vi "BS1201 Discovery Parser.vi"(10 "IP Address":string, 11 "Discovery String":string) -> (3 "Devices":T1[](array[typedef]))   [LabVIEW 2021, in "BS120x Driver.lvlib"]
uses:
  BS120x Driver.lvlib
  New BS120x Device/DiscoveredDevice.ctl
  TypeDefs/UnitType.ctl
  TypeDefs/Protocol.ctl
  BS120x.lvclass
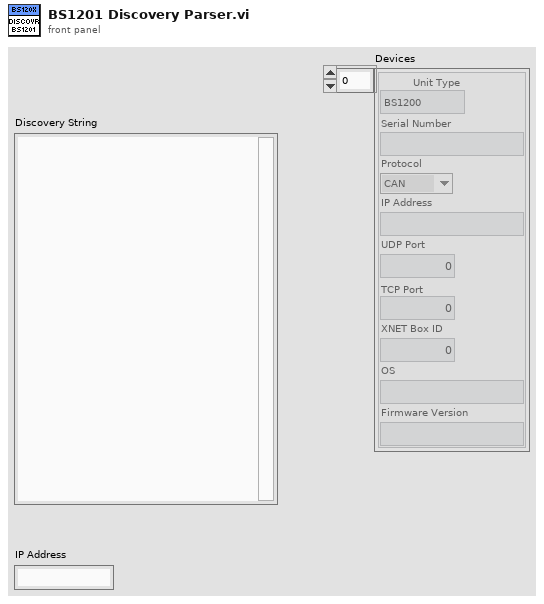
[diagram p1: front panel]
types:
  T1 = typedef "BS120x Driver.lvlib/DiscoveredDevice.ctl" = cluster{"Unit Type":T2, "Serial Number":string, "Protocol":T3, "IP Address":string, "UDP Port":u16, "TCP Port":u16, "XNET Box ID":u8, "OS":string, "Firmware Version":string}
  T2 = typedef "BS120x Driver.lvlib/BS120x.lvclass/UnitType.ctl" = enum16{"BS1200", "BS1201"}
  T3 = typedef "BS120x Driver.lvlib/BS120x.lvclass/Protocol.ctl" = enum16{"CAN", "Ethernet"}
  T4 = cluster{"IP Address":string, "SN":string, "IP Enabled":string, "UDP Port":string, "TCP Port":string, "Box ID":string}
  T5 = cluster{"IP Address":string, "SN":string, "IP Enabled":bool, "UDP Port":u16, "TCP Port":u16, "Box ID":u8}
  T6 = cluster{"[0]":string, "[1]":string, "[2]":string, "[3]":string, "[4]":string, "[5]":string}
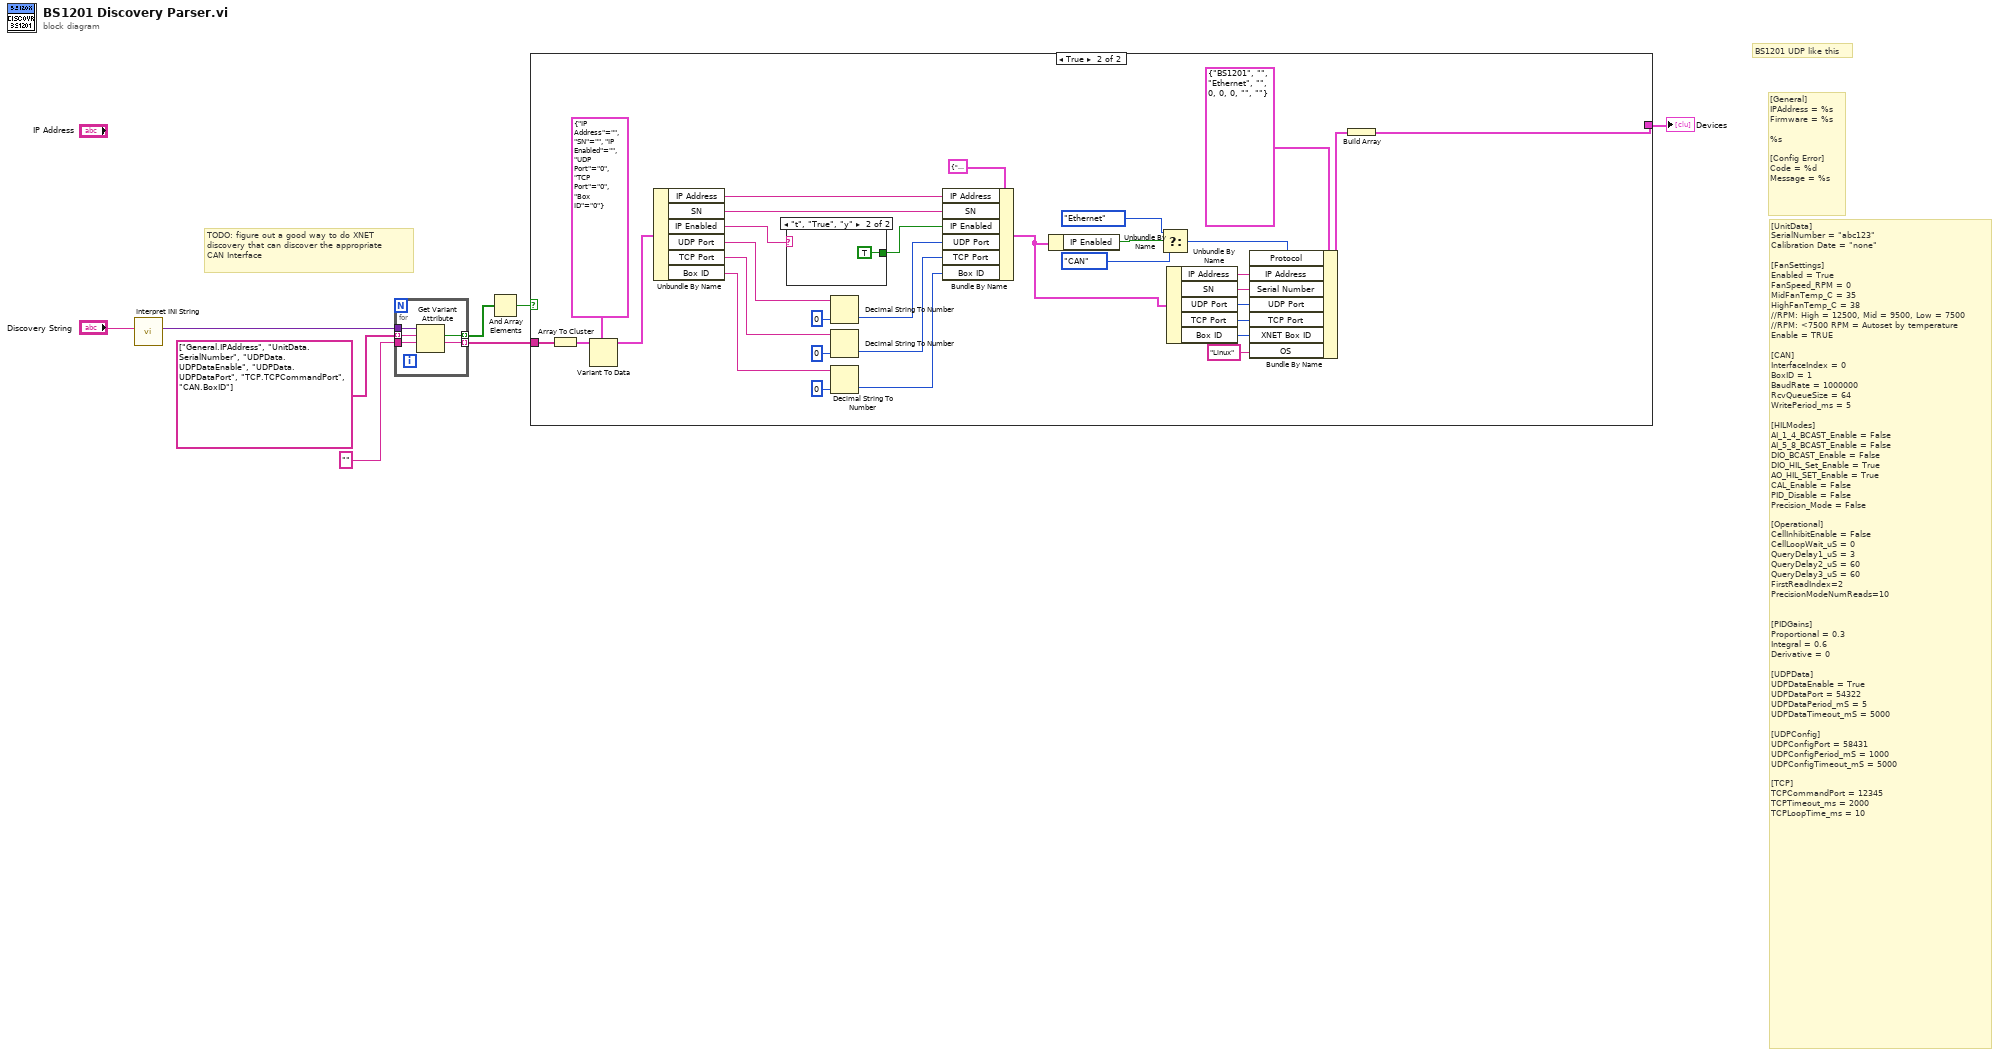
[diagram p0: block diagram]
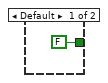
[diagram p3: hidden frame]
diagram:
  # "[UnitData]\nSerialNumber = \"abc123\"\nCalibration Date = \"none\"\n\n[FanSettings]\nEnabled = True\nFanSpeed_RPM = 0\nMidFanTemp_C = 35\nHighFanTemp_C = 38\n//RPM: High = 12500, Mid = 9500, Low = 7500\n//RPM: <7500 RPM = Autoset by temperature\nEnable = TRUE\n\n[CAN]\nInterfaceIndex = 0\nBoxID = 1\nBaudRate = 1000000\nRcvQueueSize = 64\nWritePeriod_ms = 5\n\n[HILModes]\nAI_1_4_BCAST_Enable = False\nAI_5_8_BCAST_Enable = False\nDIO_BCAST_Enable = False\nDIO_HIL_Set_Enable = True\nAO_HIL_SET_Enable = True\nCAL_Enable = False\nPID_Disable = False\nPrecision_Mode = False\n\n[Operational]\nCellInhibitEnable = False\nCellLoopWait_uS = 0\nQueryDelay1_uS = 3\nQueryDelay2_uS = 60\nQueryDelay3_uS = 60\nFirstReadIndex=2\nPrecisionModeNumReads=10\n\n\n[PIDGains]\nProportional = 0.3\nIntegral = 0.6\nDerivative = 0\n\n[UDPData]\nUDPDataEnable = True\nUDPDataPort = 54322\nUDPDataPeriod_mS = 5\nUDPDataTimeout_mS = 5000\n\n[UDPConfig]\nUDPConfigPort = 58431\nUDPConfigPeriod_mS = 1000\nUDPConfigTimeout_mS = 5000\n\n[TCP]\nTCPCommandPort = 12345\nTCPTimeout_ms = 2000\nTCPLoopTime_ms = 10"
  # "BS1201 UDP like this"
  # "[General]\nIPAddress = %s\nFirmware = %s\n\n%s\n\n[Config Error]\nCode = %d\nMessage = %s"
  # "TODO: figure out a good way to do XNET discovery that can discover the appropriate CAN Interface"
  n1 = call "Interpret INI String.vi"("INI String"="Discovery String") -> ("Config Map"=w8:variant)  [unwired: 9 in, 1 out]
  n2 = for {
    tunnel: w8 -> [w13]
    tunnel: "" -> [w12]
    tunnel: string[] ["General.IPAddress", "UnitData.SerialNumber", "UDPData.UDPDataEnable", "UDPData.UDPDataPort", "TCP.TCPCommandPort", "CAN.BoxID"] -> [w11] mode=indexing
    tunnel: [w10] -> w6 mode=indexing
    tunnel: [w9] -> w5 mode=indexing
    n3 = Get Variant Attribute(Variant=w13, name=w11, default value (empty Variant)=w12) -> (found=w9:bool, value=w10:string)  [unwired: 1 in, 2 out]
  }
  n4 = And Array Elements(Boolean array=w5) -> (logical AND=w4:bool)
  n5 = case shown="True" w4 {
    tunnel: w6 -> [_ w45]
    tunnel: [_ w14] -> w2
    frame False {
    }
    frame True {
      n6 = Array To Cluster(array=w45) -> (cluster=w44:T6)
      n7 = Variant To Data(type=T4 {"IP Address"="", "SN"="", "IP Enabled"="", "UDP Port"="0", "TCP Port"="0", "Box ID"="0"} ("Device"), Variant=w44) -> (data=w42:T4)  [unwired: 1 in, 1 out]
      n8 = Unbundle By Name(w42) -> ("IP Address"=w27:string, "SN"=w40:string, "IP Enabled"=w29:string, "UDP Port"=w38:string, "TCP Port"=w37:string, "Box ID"=w36:string)
      n9 = case shown="\"t\", \"True\", \"y\"" w29 {
        tunnel: [FALSE TRUE] -> w28
        frame Default {
        }
        frame "t", "True", "y" {
        }
      }
      n10 = Decimal String To Number(string=w38, default (0L)=u16 0 ("default (0 I32)")) -> (number=w32:u16)  [unwired: 1 in, 1 out]
      n11 = Decimal String To Number(string=w37, default (0L)=u16 0 ("default (0 I32)")) -> (number=w31:u16)  [unwired: 1 in, 1 out]
      n12 = Decimal String To Number(string=w36, default (0L)=u8 0 ("default (0 I32)")) -> (number=w30:u8)  [unwired: 1 in, 1 out]
      n13 = Bundle By Name(cluster=T5 {"IP Address"="", "SN"="", "IP Enabled"=FALSE, "UDP Port"=0, "TCP Port"=0, "Box ID"=0} ("Device"), "IP Address"=w27, "SN"=w40, "IP Enabled"=w28, "UDP Port"=w32, "TCP Port"=w31, "Box ID"=w30) -> (w39:T5)
      n14 = Unbundle By Name(w39) -> ("IP Enabled"=w18:bool)
      n15 = Select(t=Protocol."Ethernet" ("Protocol"), s=w18, f=Protocol."CAN" ("Protocol")) -> (s? t:f=w15:T3)
      n16 = Unbundle By Name(w39) -> ("IP Address"=w21:string, "SN"=w25:string, "UDP Port"=w24:u16, "TCP Port"=w23:u16, "Box ID"=w20:u8)
      n17 = Bundle By Name(cluster=T1 {"Unit Type"=enum."BS1201", "Serial Number"="", "Protocol"=enum."Ethernet", "IP Address"="", "UDP Port"=0, "TCP Port"=0, "XNET Box ID"=0, "OS"="", "Firmware Version"=""} ("Device"), "Protocol"=w15, "IP Address"=w21, "Serial Number"=w25, "UDP Port"=w24, "TCP Port"=w23, "XNET Box ID"=w20, "OS"="Linux" ("Comment")) -> (w22:T1)
      n18 = Build Array(w22) -> (w14:T1[])
    }
  }
  "Devices" <- w2
